vi "calibrate DO.vi"(11 "Index":u32) -> ()   [LabVIEW 2012]
uses:
  toolbar icons/help.ctl
  DAQ configuration/Sensor buffer command.ctl
  global scale array.vi
panel:
  in  "Help Button":T1
  in  "Ithaca atm":bool
  out "Sample Temperature":dbl[unit] format="%.1f"
  in  "Calibrate":bool
  in  "OK Button":bool
  out "name":string
  out "units":string
  in  "Temperature\nChannel":i32 min=0 step=1
  in  "Temperature\ncompensated":bool
  in  "Barometric pressure":dbl[unit]=101300.0
  out "DO":sgl[unit] format="%.1f"
  out "DO voltage":sgl[unit] format="%.1f"
  out "XY Graph":cluster{dbl[], dbl[]}[](graph)
  out "Quit":bool
  in  "Temperature":sgl[unit]=293.15 format="%.2f"
  out "DO sat (mg/L)":dbl format="%.2f"
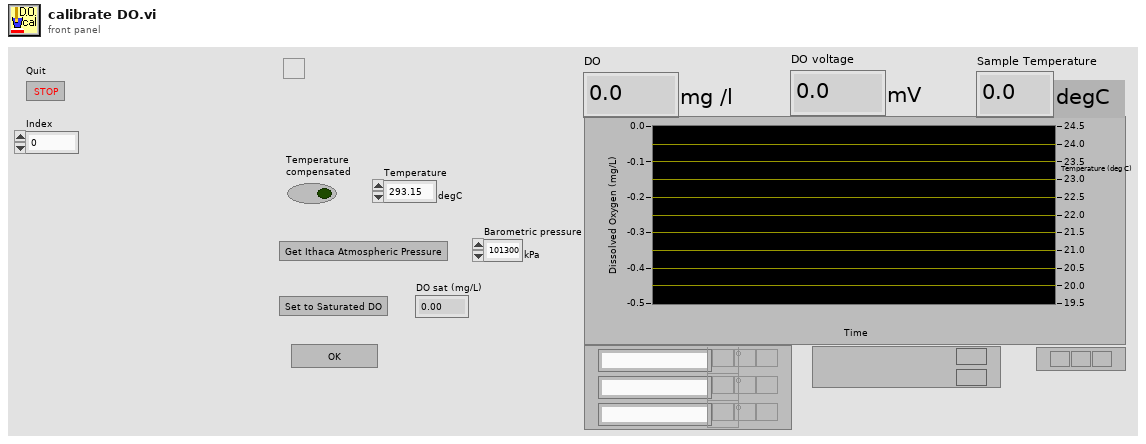
[diagram p1: front panel]
types:
  T1 = typedef "help.ctl" = bool
  T2 = typedef "Sensor buffer command.ctl" = enum16{"read average", "read recent", "read all", "write", "configure", "clear"}
  T3 = enum16{"Volts", "Polynomial", "Correspondence Table", "pH", "Dissolved Oxygen"}
  T4 = typedef "calib array.ctl" = T5[]
  T5 = typedef "conversion.ctl" = cluster{"conversion matrix":sgl[][], "units":string, "name":string, "scale type":T6, "offset (volts)":dbl, "second channel":i8, "correspondence table":T7, "offset (physical units)":dbl, "pH scale":T8, "D.O.":T9}
  T6 = typedef "scale type.ctl" = enum16{"Volts", "Polynomial", "Correspondence Table", "pH", "Dissolved Oxygen", "Quadratic"}
  T7 = typedef "correspondence table.ctl" = cluster{"physical units":dbl, "volts":dbl}[]
  T8 = typedef "pH scale.ctl" = cluster{"Buffers":cluster{"Buffer":dbl, "Calibrated":bool, "V/T":dbl}[], "Temperature":dbl}
  T9 = typedef "DO scale.ctl" = cluster{"Temperature":dbl, "K":dbl, "barometric pressure":dbl}
  T10 = typedef "Sensor data.ctl" = cluster{" Sensor array":T11[], "Time":dbl}
  T11 = typedef "sensor cluster.ctl" = cluster{"voltage":sgl, "scaled":sgl, "units":string, "Out of Range":bool}
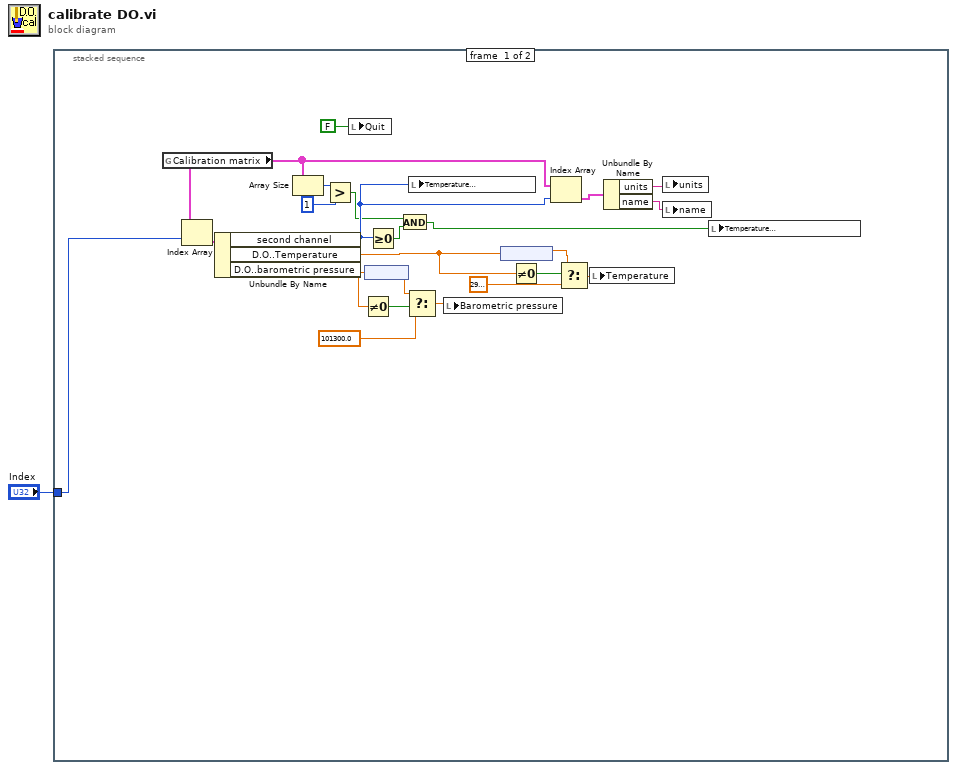
[diagram p0: block diagram]
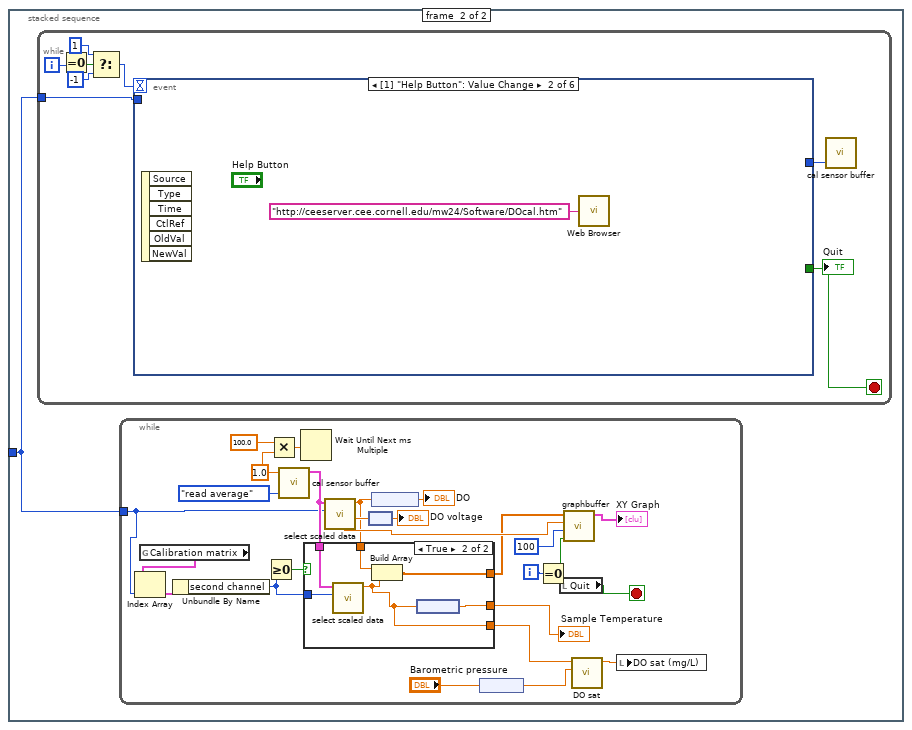
[diagram p2: hidden frame]
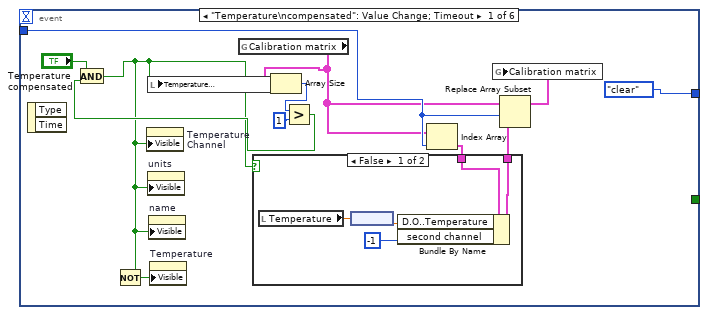
[diagram p3: hidden frame]
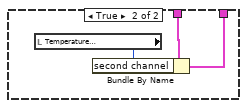
[diagram p4: hidden frame]
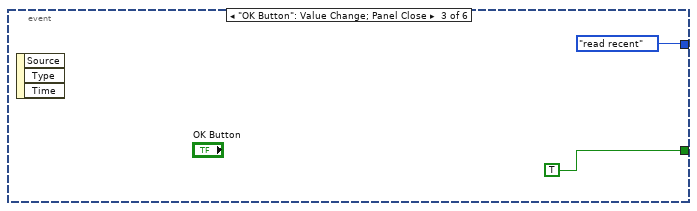
[diagram p5: hidden frame]
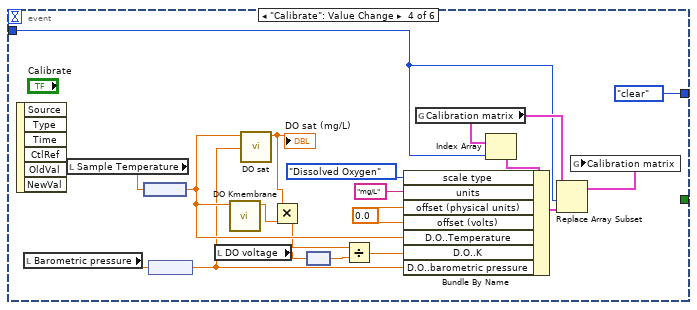
[diagram p6: hidden frame]
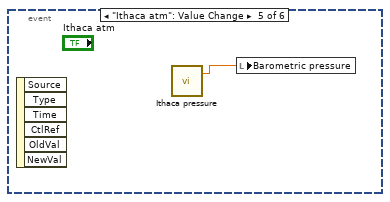
[diagram p7: hidden frame]
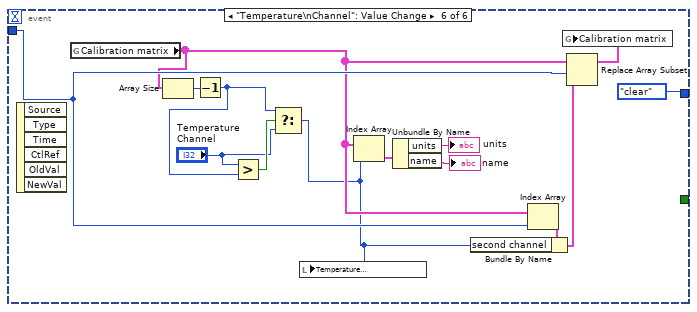
[diagram p8: hidden frame]
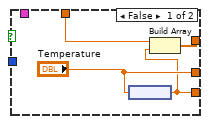
[diagram p9: hidden frame]
diagram:
  n1 = stacked-sequence {
    tunnel: "Index" -> [w22 w25]
    frame #0 {
      n2 = global read "global scale array.vi" "Calibration matrix"() -> (w8:T4)
      n3 = Index Array(array=w8, index=w22) -> (element=w24:T5)
      n4 = Unbundle By Name(w24) -> ("second channel"=w19:i8, "D.O..Temperature"=w13:dbl, "D.O..barometric pressure"=w15:dbl)
      n5 = Array Size(array=w8) -> (size(s)=w7:i32)
      n6 = Greater?(x=w7, y=1) -> (0:w5:bool)
      n7 = local write "Quit"(FALSE ("Quit")) -> ()
      n8 = Not Equal To 0?(x=w15) -> (x != 0?=w14:bool)
      n9 = node(w15) -> (w16:dbl[unit])
      n10 = Greater Or Equal To 0?(x=w19) -> (x >= 0?=w4:bool)
      n11 = And(x=w5, y=w4) -> (x .and. y?=w3:bool)
      n12 = Select(t=w16, s=w14, f=dbl[unit] 101300.0) -> (s? t:f=w17:dbl[unit])
      n13 = local write "Temperature\nChannel"(w19) -> ()
      n14 = local write "Barometric pressure"(w17) -> ()
      n15 = node(w13) -> (w12:dbl[unit])
      n16 = Not Equal To 0?(x=w13) -> (x != 0?=w10:bool)
      n17 = Index Array(array=w8, index=w19) -> (element=w23:T5)
      n18 = Select(t=w12, s=w10, f=dbl[unit] 295.15) -> (s? t:f=w11:dbl[unit])
      n19 = local write "Temperature"(w11) -> ()
      n20 = Unbundle By Name(w23) -> ("units"=w20:string, "name"=w21:string)
      n21 = local write "units"(w20) -> ()
      n22 = local write "name"(w21) -> ()
      n23 = local write "Temperature\ncompensated"(w3) -> ()
    }
    frame #1 {
      n24 = while {
        tunnel: w25 -> [w33]
        i -> [w28]
        stop <- w32 stop-if-true
        n25 = Equal To 0?(x=w28) -> (x = 0?=w27:bool)
        n26 = Select(t=1, s=w27, f=-1) -> (s? t:f=w31:i32)
        n27 = event shown="[1] \"Help Button\": Value Change" {
          selector: _ -> [_ _ _ _ _ _]
          dyn-events: _ -> [_ _ _ _ _ _]
          timeout: w31 -> [_ _ _ _ _ _]
          tunnel: w33 -> [w42 _ _ w61 _ w84]
          tunnel: [_ _ TRUE ("OK Button") _ _ _] -> w32
          tunnel: [Sensor_buffer_command."clear" ("command") _ Sensor_buffer_command."read recent" ("command") Sensor_buffer_command."clear" ("command") _ Sensor_buffer_command."clear" ("command")] -> w26
          event "Temperature\ncompensated": Value Change; Timeout {
            n28 = event-data() -> ()  [unwired: 1 in, 2 out]
            n29 = global read "global scale array.vi" "Calibration matrix"() -> (w39:T4)
            n30 = Array Size(array=w39) -> (size(s)=w38:i32)
            n31 = Greater?(x=w38, y=1) -> (0:w36:bool)
            n32 = And(x="Temperature\ncompensated", y=w36) -> (x .and. y?=w34:bool)
            n33 = Not(x=w34) -> (.not. x?=w41:bool)
            n34 = property on="Temperature\nChannel" class="DigNum (strict)"("Visible"=w34) -> ()  [unwired: 2 in, 2 out]
            n35 = local write "Temperature\ncompensated"(w34) -> ()
            n36 = property on="units" class="Str"("Visible"=w34) -> ()  [unwired: 2 in, 2 out]
            n37 = property on="name" class="Str"("Visible"=w34) -> ()  [unwired: 2 in, 2 out]
            n38 = property on="Temperature" class="DigNum (strict)"("Visible"=w41) -> ()  [unwired: 2 in, 2 out]
            n39 = Index Array(array=w39, index=w42) -> (element=w44:T5)
            n40 = case shown="False" w34 {
              tunnel: w44 -> [w50 w52]
              tunnel: [w49 w51] -> w43
              frame False {
                n41 = local read "Temperature"() -> (w47:sgl[unit])
                n42 = node(w47) -> (w46:sgl)
                n43 = Bundle By Name(cluster=w50, "D.O..Temperature"=w46, "second channel"=i8 -1) -> (w49:T5)
              }
              frame True {
                n44 = local read "Temperature\nChannel"() -> (w53:i32)
                n45 = Bundle By Name(cluster=w52, "second channel"=w53) -> (w51:T5)
              }
            }
            n46 = Replace Array Subset(array=w39, new element=w43, index=w42) -> (w45:T4)
            n47 = global write "global scale array.vi" "Calibration matrix"(w45) -> ()
          }
          event Value Change {
            n48 = event-data() -> ()  [unwired: 1 in, 6 out]
            n49 = call "Web Browser.vi"("URL"="http://ceeserver.cee.cornell.edu/mw24/Software/DOcal.htm") -> ()  [unwired: 1 in]
          }
          event "OK Button": Value Change; Panel Close {
            n50 = event-data() -> ()  [unwired: 1 in, 3 out]
          }
          event "Calibrate": Value Change {
            w67 = 0.0 ("offset (physical units)")
            n51 = event-data() -> ()  [unwired: 1 in, 6 out]
            n52 = local read "Barometric pressure"() -> (w73:dbl[unit])
            n53 = local read "Sample Temperature"() -> (w74:dbl[unit])
            n54 = node(w74) -> (w75:dbl)
            n55 = node(w73) -> (w57:dbl)
            n56 = local read "DO voltage"() -> (w60:sgl[unit])
            n57 = call "DO Kmembrane.vi"("Temperature (C)"=w75) -> ("Kmembrane"=w62:dbl)  [unwired: 10 in]
            n58 = call "DO sat.vi"("Atmospheric Pressure (kPa)"=w57, "Temperature (C)"=w75) -> ("DO sat (mg/L)"=w64:dbl)  [unwired: 9 in]
            "DO sat (mg/L)" <- w64
            n59 = Multiply(x=w64, y=w62) -> (x*y=w63:dbl)
            n60 = node(w60) -> (w59:sgl)
            n61 = Divide(x=w63, y=w59) -> (x/y=w68:dbl)
            n62 = global read "global scale array.vi" "Calibration matrix"() -> (w72:T4)
            n63 = Index Array(array=w72, index=w61) -> (element=w69:T5)
            n64 = Bundle By Name(cluster=w69, "scale type"=T3."Dissolved Oxygen", "units"="mg/L", "offset (physical units)"=w67, "offset (volts)"=w67, "D.O..Temperature"=w75, "D.O..K"=w68, "D.O..barometric pressure"=w57) -> (w71:T5)
            n65 = Replace Array Subset(array=w72, new element=w71, index=w61) -> (w70:T4)
            n66 = global write "global scale array.vi" "Calibration matrix"(w70) -> ()
          }
          event "Ithaca atm": Value Change {
            n67 = event-data() -> ()  [unwired: 1 in, 6 out]
            n68 = call "Ithaca pressure.vi"() -> ("Atmospheric pressure"=w76:dbl[unit])  [unwired: 1 in, 1 out]
            n69 = local write "Barometric pressure"(w76) -> ()
          }
          event "Temperature\nChannel": Value Change {
            n70 = event-data() -> ()  [unwired: 1 in, 6 out]
            n71 = global read "global scale array.vi" "Calibration matrix"() -> (w80:T4)
            n72 = Array Size(array=w80) -> (size(s)=w83:i32)
            n73 = Decrement(x=w83) -> (x-1=w81:i32)
            n74 = Greater?(x="Temperature\nChannel", y=w81) -> (0:w82:bool)
            n75 = Select(t=w81, s=w82, f="Temperature\nChannel") -> (s? t:f=w78:i32)
            n76 = local write "Temperature\nChannel"(w78) -> ()
            n77 = Index Array(array=w80, index=w78) -> (element=w90:T5)
            n78 = Unbundle By Name(w90) -> ("units"=→"units":string, "name"=→"name":string)
            n79 = Index Array(array=w80, index=w84) -> (element=w88:T5)
            n80 = Bundle By Name(cluster=w88, "second channel"=w78) -> (w87:T5)
            n81 = Replace Array Subset(array=w80, new element=w87, index=w84) -> (w89:T4)
            n82 = global write "global scale array.vi" "Calibration matrix"(w89) -> ()
          }
        }
        "Quit" <- w32
        n83 = call "cal sensor buffer.vi"("command"=w26) -> ()  [unwired: 4 in, 3 out]
      }
      n84 = while {
        tunnel: w25 -> [w98]
        i -> [w109]
        stop <- w116 stop-if-true
        w112 = sgl 1.0 ("smooth interval (s)")
        n85 = global read "global scale array.vi" "Calibration matrix"() -> (w104:T4)
        n86 = Index Array(array=w104, index=w98) -> (element=w103:T5)
        n87 = Unbundle By Name(w103) -> ("second channel"=w102:i8)
        n88 = Greater Or Equal To 0?(x=w102) -> (x >= 0?=w101:bool)
        n89 = Multiply(x=100.0 ("y"), y=w112) -> (x*y=w114:dbl)
        n90 = call "cal sensor buffer.vi"("command"=Sensor_buffer_command."read average", "smooth interval (s)"=w112) -> ("Sensor Data smoothed"=w100:T10)  [unwired: 3 in, 2 out]
        n91 = Wait Until Next ms Multiple(millisecond multiple=w114) -> ()  [unwired: 1 out]
        n92 = call "select scaled data.vi"("Sensor index"=w98, "Sensor Data"=w100) -> ("voltage"=w105:sgl, "scaled"=w97:sgl, "Time"=w111:dbl)  [unwired: 4 in, 3 out]
        n93 = case shown="True" w101 {
          tunnel: w100 -> [_ w126]
          tunnel: w102 -> [_ w125]
          tunnel: w97 -> [w120 w124]
          tunnel: [w119 w123] -> w99
          tunnel: ["Temperature" w122] -> w94
          tunnel: [w117 w121] -> w93
          frame False {
            n94 = node("Temperature") -> (w117:sgl)
            n95 = Build Array(w120, w117) -> (w119:sgl[])
          }
          frame True {
            n96 = call "select scaled data.vi"("Sensor index"=w125, "Sensor Data"=w126) -> ("scaled"=w121:sgl)  [unwired: 4 in, 5 out]
            n97 = Build Array(w124, w121) -> (w123:sgl[])
            n98 = node(w121) -> (w122:sgl[unit])
          }
        }
        "Sample Temperature" <- w94
        n99 = node(w105) -> (→"DO voltage":sgl[unit])
        n100 = node(w97) -> (→"DO":sgl[unit])
        n101 = node("Barometric pressure") -> (w91:dbl)
        n102 = Equal To 0?(x=w109) -> (x = 0?=w108:bool)
        n103 = local read "Quit"() -> (w116:bool)
        n104 = call "graphbuffer.vi"("Reset"=w108, "history length"=u16 100, "Time"=w111, "data"=w99) -> ("Multiplot graph data"=→"XY Graph":cluster{dbl[], dbl[]}[])  [unwired: 5 in, 2 out]
        n105 = call "DO sat.vi"("Atmospheric Pressure (kPa)"=w91, "Temperature (C)"=w93) -> ("DO sat (mg/L)"=w95:dbl)  [unwired: 9 in]
        n106 = local write "DO sat (mg/L)"(w95) -> ()
      }
    }
  }
